vi "动作测试.vi"() -> ()   [LabVIEW 2016]
uses:
  <vilib>/myRIO/Instrument Drivers/Onboard IO/PWM/typedefs/PWM Reference.ctl
  <vilib>/myRIO/Common/Instrument Driver Framework/Utilities/typedefs/myRIO Generic Hardware Reference.ctl
  <vilib>/myRIO/Common/Instrument Driver Framework/Utilities/typedefs/Hardware Version Enum.ctl
  <vilib>/myRIO/Common/Instrument Driver Framework/Utilities/typedefs/myRIO v1.0 Reference.ctl
  <vilib>/myRIO/Common/Instrument Driver Framework/Utilities/typedefs/Generic FPGA Reference.ctl
  <vilib>/myRIO/Common/Instrument Driver Framework/myRIO v1.0/PWM/typedefs/PWM Channels Enum.ctl
  <vilib>/myRIO/Instrument Drivers/Onboard IO/PWM/typedefs/PWM Configuration.ctl
  <vilib>/userdefined/High Color/nirio_resource_hc.ctl
  <vilib>/myRIO/Instrument Drivers/Onboard IO/DIO/typedefs/DIO Reference.ctl
  <vilib>/myRIO/Common/Instrument Driver Framework/myRIO v1.0/DIO/typedefs/DIO Channels List.ctl
  <vilib>/myRIO/Common/Instrument Driver Framework/myRIO v1.0/DIO/typedefs/DIO Channels Enum.ctl
  <vilib>/myRIO/Common/Instrument Driver Framework/Utilities/vis/Is FPGA Ref Available.vi
  <vilib>/myRIO/Common/Instrument Driver Framework/myRIO v1.0/DIO/vis/myRIO v1.1 Open DIO.vi
  <vilib>/myRIO/Instrument Drivers/Onboard IO/DIO/vis/Write.vi
  <vilib>/myRIO/Common/Instrument Driver Framework/myRIO v1.0/PWM/vis/myRIO v1.1 Open PWM.vi
  <vilib>/myRIO/Instrument Drivers/Onboard IO/PWM/vis/Set Duty Cycle and Frequency.vi
  <vilib>/myRIO/Common/Instrument Driver Framework/Utilities/vis/Validate Channels.vi
  <vilib>/myRIO/Common/Instrument Driver Framework/myRIO v1.0/DIO/vis/myRIO v1.0 Reserve DIO.vi
  <vilib>/myRIO/Common/Instrument Driver Framework/myRIO v1.0/PWM/vis/myRIO v1.0 Reserve PWM.vi
  <vilib>/myRIO/Common/Instrument Driver Framework/myRIO v1.0/Resource Manager/vis/myRIO v1.0 Reserve Channel List.vi
  <vilib>/myRIO/Common/Instrument Driver Framework/myRIO v1.0/DIO/vis/myRIO v1.0 Build MUX Configuration DIO.vi
  <vilib>/myRIO/Common/Instrument Driver Framework/myRIO v1.0/PWM/vis/myRIO v1.0 Build MUX Configuration PWM.vi
  <vilib>/myRIO/Common/Instrument Driver Framework/myRIO v1.0/Resource Manager/vis/myRIO v1.0 Reserve Channel.vi
  <vilib>/myRIO/Common/Instrument Driver Framework/myRIO v1.0/Resource Manager/vis/myRIO v1.0 Unreserve Channel.vi
  <vilib>/myRIO/Common/Instrument Driver Framework/myRIO v1.0/Resource Manager/vis/myRIO v1.0 Create Configuration List.vi
  <vilib>/myRIO/Common/Instrument Driver Framework/myRIO v1.0/Resource Manager/vis/myRIO v1.0 Build Mutex Name.vi
  <vilib>/Utility/VariantDataType/GetNumericInfo.vi
  <vilib>/Utility/error.llb/Error Cluster From Error Code.vi
  <vilib>/myRIO/Common/Instrument Driver Framework/myRIO v1.0/myRIO v1.1 Open.vi
  <vilib>/myRIO/Common/Instrument Driver Framework/Utilities/vis/IO Manager.vi
  <vilib>/myRIO/Common/Instrument Driver Framework/Utilities/vis/Configuration Manager.vi
  <vilib>/myRIO/Common/Instrument Driver Framework/myRIO v1.0/Resource Manager/vis/myRIO v1.0 Configure IO.vi
  <vilib>/myRIO/Common/Instrument Driver Framework/myRIO v1.0/myRIO v1.0 Close.vi
  <vilib>/myRIO/Common/Instrument Driver Framework/myRIO v1.0/PWM/vis/myRIO v1.0 Write PWM.vi
  <vilib>/myRIO/Common/Instrument Driver Framework/myRIO v1.0/DIO/vis/myRIO v1.0 Write DIO.vi
  <vilib>/myRIO/Express VI/Onboard IO/PWM/PWM Express VI.xnode
  <vilib>/myRIO/Instrument Drivers/Onboard IO/PWM/vis/myRIO PWM Open.xnode
  <vilib>/myRIO/Express VI/Onboard IO/DO/DO Express VI.xnode
  <vilib>/myRIO/Instrument Drivers/Onboard IO/DIO/vis/myRIO DIO Open.xnode
  <vilib>/myRIO/Instrument Drivers/Onboard IO/PWM/PWM.lvlib
  <vilib>/myRIO/Instrument Drivers/Onboard IO/DIO/DIO.lvlib
panel:
  in  "后退":bool
  in  "前进":bool
  in  "手模式":enum16{"正常（手）", "同向联动（手）", "反向联动（手）"}(ring)
  in  "肘模式":enum16{"正常（肘）", "同向联动（肘）", "反向联动（肘）"}(ring)
  in  "肩模式":enum16{"正常（肩）", "同向联动（肩）", "反向联动（肩）"}(ring)
  in  "右肘":dbl(knob) scale=0.025..0.125
  in  "右肩":dbl(knob) scale=0.025..0.125
  in  "右手":dbl(knob) scale=0.025..0.125
  in  "左手":dbl(knob) scale=0.025..0.125
  in  "左肘":dbl(knob) scale=0.025..0.125
  in  "左肩":dbl(knob) scale=0.025..0.125
  in  "停止按钮":bool
  in  "左2右1":bool
  in  "左1右2":bool
  # "放"
  # "收"
  # "收"
  # "放"
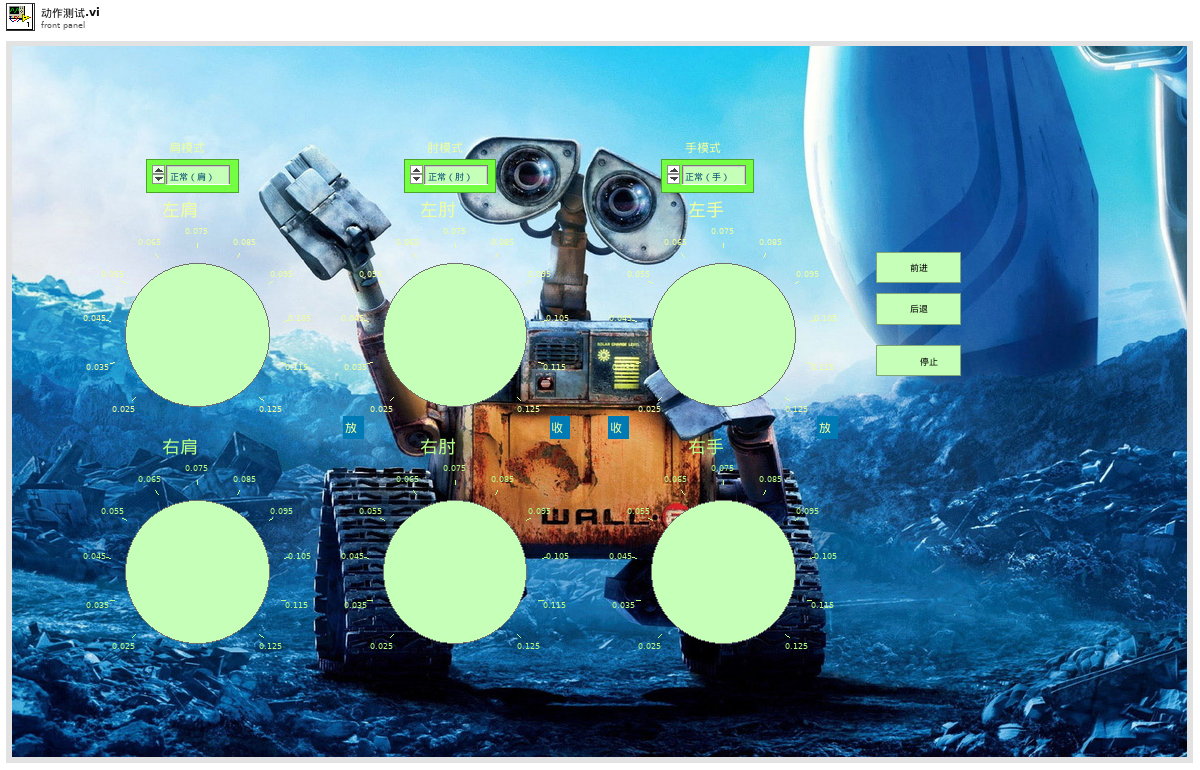
[diagram p1: front panel]
types:
  T1 = typedef "PWM.lvlib/PWM Reference.ctl" = cluster{"myRIO Reference":T2, "PWM Channels Enum":T6, "PWM Configuration":T7}
  T2 = typedef "myRIO Generic Hardware Reference.ctl" = cluster{"myRIO Model":T3, "myRIO Hardware Reference":T4}
  T3 = typedef "Hardware Version Enum.ctl" = enum16{"Unknown", "myRIO-1900", "myRIO-1950", "roboRIO", "NI ELVIS RIO CM"}
  T4 = typedef "myRIO v1.0 Reference.ctl" = cluster{"Generic FPGA Reference":T5, "Allow multiple opens":bool}
  T5 = typedef "Generic FPGA Reference.ctl" = refnum<k20>
  T6 = typedef "PWM Channels Enum.ctl" = enum16{"Not Connected", "C/PWM0", "C/PWM1", "A/PWM0", "A/PWM1", "A/PWM2", "B/PWM0", "B/PWM1", "B/PWM2", "PWM/PWM0", "PWM/PWM1", "PWM/PWM2", "PWM/PWM3", "PWM/PWM4", "PWM/PWM5", "PWM/PWM6", "PWM/PWM7", "PWM/PWM8", "PWM/PWM9"}
  T7 = typedef "PWM.lvlib/PWM Configuration.ctl" = cluster{"Frequency":dbl, "Duty Cycle":dbl}
  T8 = typedef "nirio_resource_hc.ctl" = tag
  T9 = typedef "DIO.lvlib/DIO Reference.ctl" = cluster{"myRIO Reference":T2, "DIO Channels List":T10}
  T10 = typedef "DIO Channels List.ctl" = T11[]
  T11 = typedef "DIO Channels Enum.ctl" = enum16{"Not Connected", "C/DIO0", "C/DIO1", "C/DIO2", "C/DIO3", "C/DIO4", "C/DIO5", "C/DIO6", "C/DIO7", "A/DIO0", "A/DIO1", "A/DIO2", "A/DIO3", "A/DIO4", "A/DIO5", "A/DIO6", "A/DIO7", "A/DIO8", "A/DIO9", "A/DIO10", "A/DIO11", "A/DIO12", "A/DIO13", "A/DIO14", "A/DIO15", "B/DIO0", "B/DIO1", "B/DIO2", "B/DIO3", "B/DIO4", "B/DIO5", "B/DIO6", "B/DIO7", "B/DIO8", "B/DIO9", "B/DIO10", "B/DIO11", "B/DIO12", "B/DIO13", "B/DIO14", "B/DIO15", "LED0", "LED1", "LED2", "LED3", "Button0", "DIO/DIO0", "DIO/DIO1", "DIO/DIO2", "DIO/DIO3", "DIO/DIO4", "DIO/DIO5", "DIO/DIO6", "DIO/DIO7", "DIO/DIO8", "DIO/DIO9", "SPI/CS0", "SPI/CS1", "SPI/CS2", "SPI/CS3", "LED RADIO (Green)", "LED RADIO (Red)", "LED COMM (Green)", "LED COMM (Red)", "LED MODE (Green)", "LED MODE (Red)"}
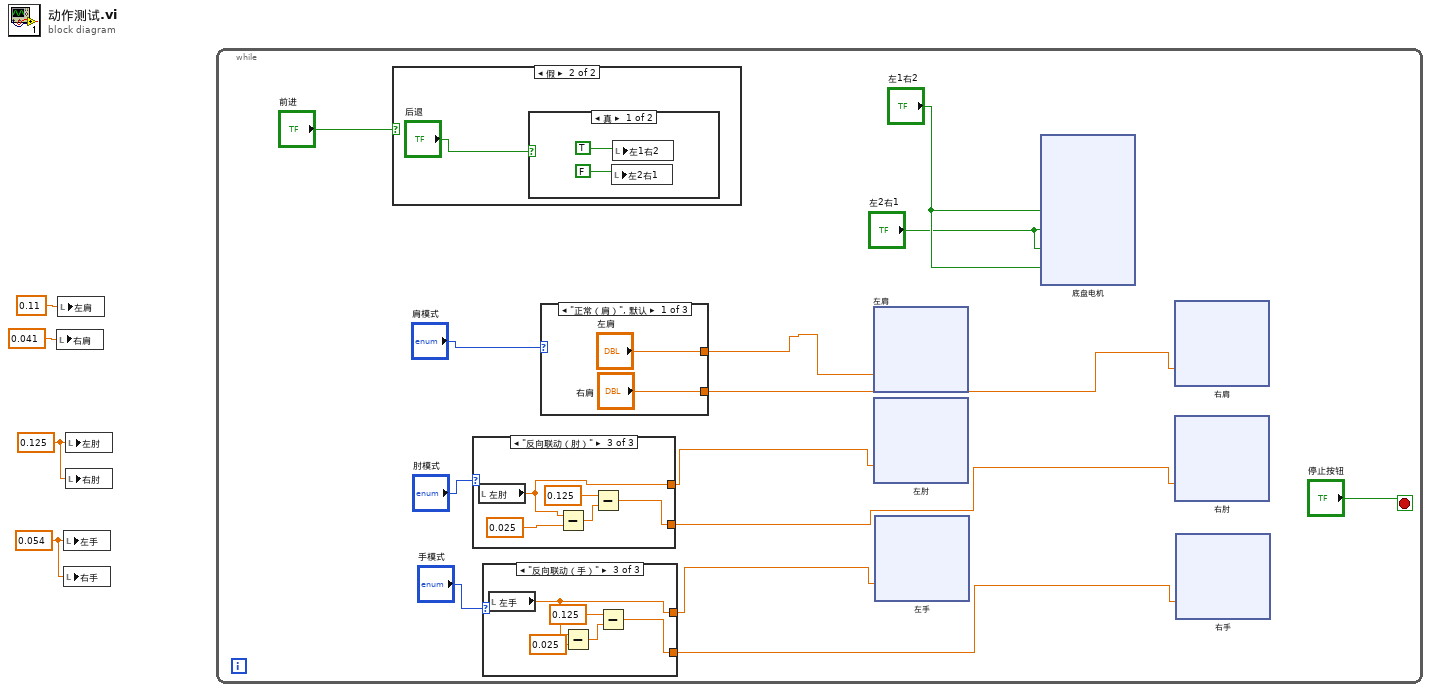
[diagram p0: block diagram]
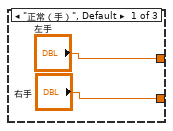
[diagram p2: hidden frame]
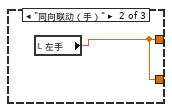
[diagram p3: hidden frame]
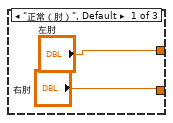
[diagram p4: hidden frame]
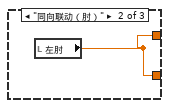
[diagram p5: hidden frame]
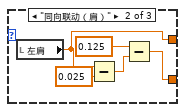
[diagram p6: hidden frame]
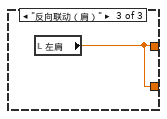
[diagram p7: hidden frame]
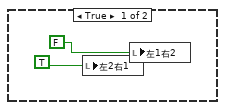
[diagram p8: hidden frame]
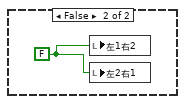
[diagram p9: hidden frame]
diagram:
  w1 = 0.054 ("左手")
  w2 = 0.125 ("左肘")
  n1 = local write "右肩"(0.041 ("右肩")) -> ()
  n2 = local write "左肩"(0.11 ("左肩")) -> ()
  n3 = local write "左手"(w1) -> ()
  n4 = local write "右手"(w1) -> ()
  n5 = local write "左肘"(w2) -> ()
  n6 = local write "右肘"(w2) -> ()
  n7 = while {
    stop <- "停止按钮" stop-if-true
    n8 = case shown="假" "前进" {
      frame True {
        n9 = local write "左2右1"(TRUE) -> ()
        n10 = local write "左1右2"(FALSE) -> ()
      }
      frame False {
        n11 = case shown="真" "后退" {
          frame True {
            n12 = local write "左2右1"(FALSE) -> ()
            n13 = local write "左1右2"(TRUE) -> ()
          }
          frame False {
            w47 = FALSE
            n14 = local write "左1右2"(w47) -> ()
            n15 = local write "左2右1"(w47) -> ()
          }
        }
      }
    }
    n16 = case shown="\"反向联动（肘）\"" "肘模式" {
      tunnel: ["左肘" w28 w29] -> w12
      tunnel: ["右肘" w28 w31] -> w11
      frame "正常（肘）", Default {
      }
      frame "同向联动（肘）" {
        n17 = local read "左肘"() -> (w28:dbl)
      }
      frame "反向联动（肘）" {
        n18 = local read "左肘"() -> (w29:dbl)
        n19 = Subtract(x=w29, y=0.025) -> (x-y=w32:dbl)
        n20 = Subtract(x=0.125, y=w32) -> (x-y=w31:dbl)
      }
    }
    n21 = case shown="\"反向联动（手）\"" "手模式" {
      tunnel: ["左手" w20 w21] -> w9
      tunnel: ["右手" w20 w22] -> w8
      frame "正常（手）", Default {
      }
      frame "同向联动（手）" {
        n22 = local read "左手"() -> (w20:dbl)
      }
      frame "反向联动（手）" {
        n23 = local read "左手"() -> (w21:dbl)
        n24 = Subtract(x=w21, y=0.025) -> (x-y=w24:dbl)
        n25 = Subtract(x=0.125, y=w24) -> (x-y=w22:dbl)
      }
    }
    n26 = case shown="\"正常（肩）\", 默认" "肩模式" {
      tunnel: ["左肩" w36 w41] -> w15
      tunnel: ["右肩" w37 w41] -> w14
      frame "正常（肩）", Default {
      }
      frame "同向联动（肩）" {
        n27 = local read "左肩"() -> (w36:dbl)
        n28 = Subtract(x=w36, y=0.025) -> (x-y=w39:dbl)
        n29 = Subtract(x=0.125, y=w39) -> (x-y=w37:dbl)
      }
      frame "反向联动（肩）" {
        n30 = local read "左肩"() -> (w41:dbl)
      }
    }
    n31 = xnode "左肩"("Duty Cycle"=w15) -> ()  [unwired: 1 in, 1 out]
    n32 = xnode "左肘"("Duty Cycle"=w12) -> ()  [unwired: 1 in, 1 out]
    n33 = xnode "左手"("Duty Cycle"=w9) -> ()  [unwired: 1 in, 1 out]
    n34 = xnode "底盘电机"("Left Out 1 (C/DIO0 (DIO0))"="左1右2", "Left Out 2 (C/DIO1 (DIO1))"="左2右1", "Right Out 1 (C/DIO2 (DIO2))"="左2右1", "Right Out 2 (C/DIO3 (DIO3))"="左1右2") -> ()  [unwired: 1 in, 1 out]
    n35 = xnode "右肩"("Duty Cycle"=w14) -> ()  [unwired: 1 in, 1 out]
    n36 = xnode "右肘"("Duty Cycle"=w11) -> ()  [unwired: 1 in, 1 out]
    n37 = xnode "右手"("Duty Cycle"=w8) -> ()  [unwired: 1 in, 1 out]
  }
